vi "FormatThreadedCall.vi"(1 "executor":string="executor", 2 "thread #":i32, 3 "call":string) -> (0 "python object":string)   [LabVIEW 2014, in "Raspberry Pi Compatible Compiler for LabVIEW.lvlib" / "Python Functions.lvlib"]
uses:
  Python Functions.lvlib
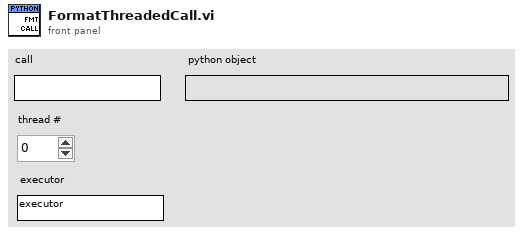
[diagram p1: front panel]
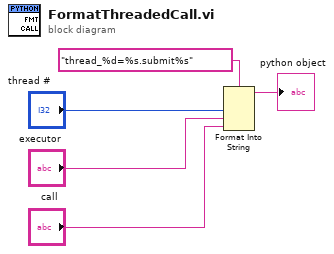
[diagram p0: block diagram]
diagram:
  n1 = Format Into String(format string="thread_%d=%s.submit%s", "thread #", "executor", "call") -> (resulting string=→"python object":string)  [unwired: 2 in, 1 out]
